vi "ErrorCheck.vi"(4 "Base Error (0)":i32, 5 "payload":string, 6 "error in":errorcluster) -> (0 "error out":errorcluster)   [LabVIEW 2014, in "RasPiDownloader.lvlib"]
uses:
  RasPiDownloader.lvlib
  ErrorMessageTD.ctl
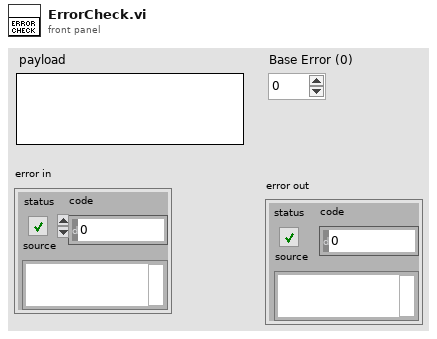
[diagram p1: front panel]
types:
  T1 = typedef "RasPiDownloader.lvlib/ErrorMessageTD.ctl" = cluster{"error":i32, "error_msg":string}
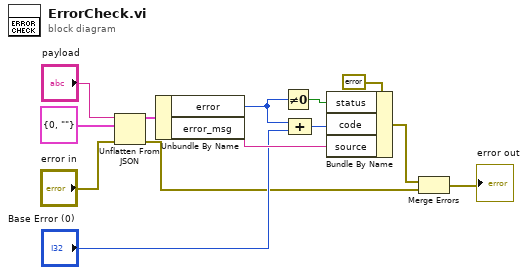
[diagram p0: block diagram]
diagram:
  n1 = Unflatten From JSON(JSON string="payload", type and defaults=T1 {"error"=0, "error_msg"=""} ("error"), error in (no error)="error in") -> (value=w12:T1, error out=w5:errorcluster)  [unwired: 4 in]
  n2 = Unbundle By Name(w12) -> ("error"=w8:i32, "error_msg"=w10:string)
  n3 = Not Equal To 0?(x=w8) -> (x != 0?=w7:bool)
  n4 = Compound Arithmetic op=ADD(w8, "Base Error (0)") -> (w9:i32)
  n5 = Bundle By Name(cluster=errorcluster {"status"=FALSE, "code"=0, "source"=""} ("error constant"), "status"=w7, "code"=w9, "source"=w10) -> (w4:errorcluster)
  n6 = Merge Errors(w4, w5) -> (→"error out":errorcluster)
